vi "Init.vi"(8 "error in (no error)":errorcluster, 10 "Connection String":string, 11 "Camera in":refnum<class "CameraI2COUSB.lvclass">) -> (0 "error out":errorcluster, 3 "Camera out":refnum<class "CameraI2COUSB.lvclass">)   [LabVIEW 2020, in "CameraI2COUSB.lvlib" / "CameraI2COUSB.lvclass"]
doc: "Inizialize camera object\n\n<b> ConnectionString:</b> String with parameters needed to connecting to camera. The parameters are separate by ::\nThe format is: <Vid>::<Pid>::<Device Index>::<Clock Rate>::<Provider Name>"
uses:
  CameraI2COUSB.lvclass
  Private/TypeDef/Init_FSMDate.ctl
  Private/TypeDef/Init_Step.ctl
  CameraI2COUSB.lvclass/CameraI2COUSB.ctl
  <vilib>/Utility/error.llb/Error Cluster From Error Code.vi
  <vilib>/Utility/LVClass/Get LV Class Default Value.vi
  <vilib>/ErrorRing/Error Ring.xnode
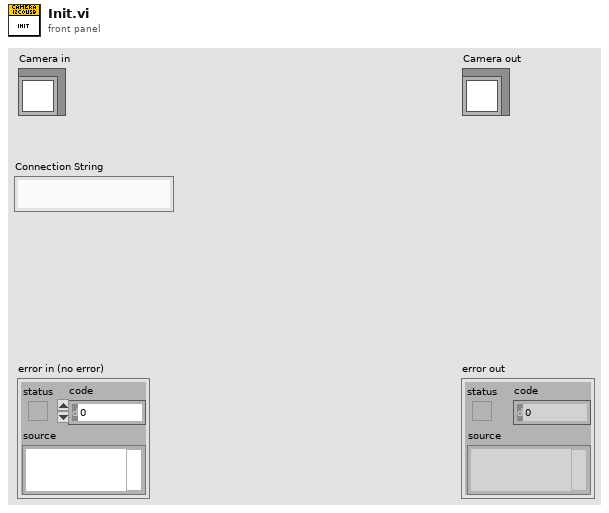
[diagram p1: front panel]
types:
  T1 = typedef "CameraI2COUSB.lvlib/CameraI2COUSB.lvclass/Init_FSMDate.ctl" = cluster{"States":T2[], "PrjctItemRef":refnum<vi>}
  T2 = typedef "CameraI2COUSB.lvlib/CameraI2COUSB.lvclass/Init_Step.ctl" = enum16{"AcquireConnPrms", "SetConfigParams", "CheckDriverFolder", "FindDriverClass", "LoadDriver", "Map Cmds to Registers", "Create Events"}
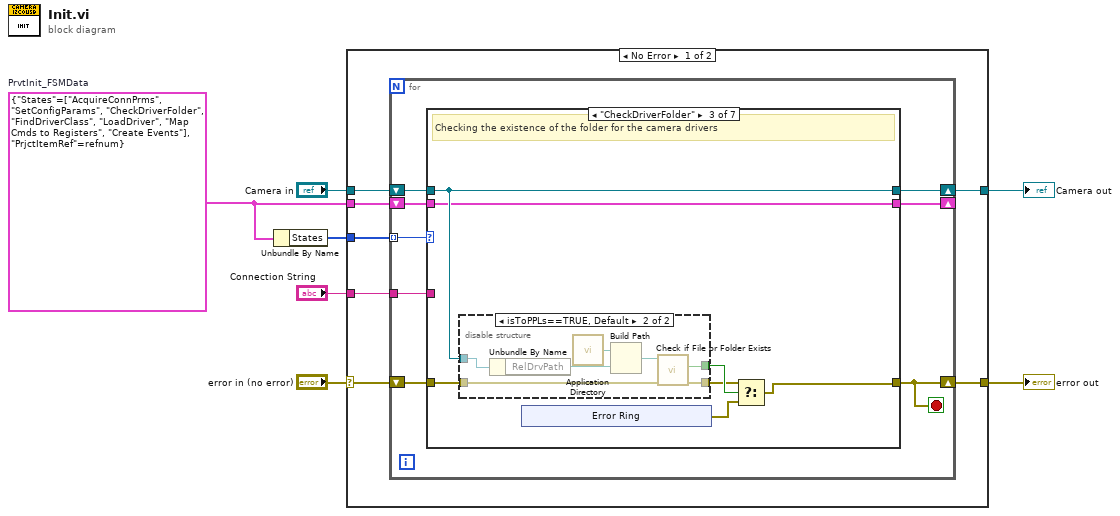
[diagram p0: block diagram]
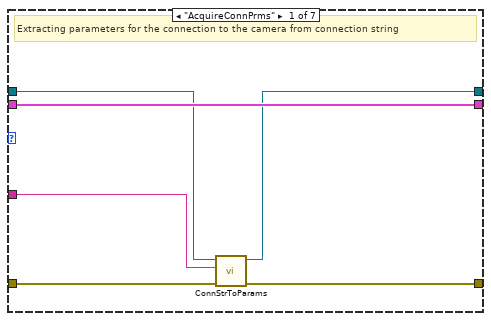
[diagram p2: hidden frame]
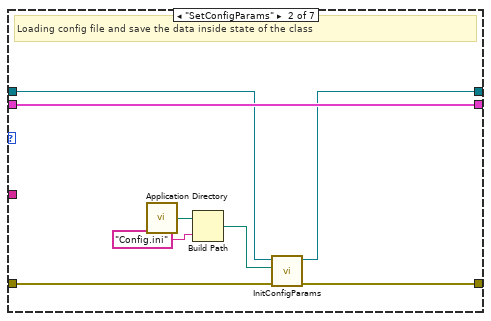
[diagram p3: hidden frame]
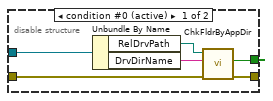
[diagram p4: hidden frame]
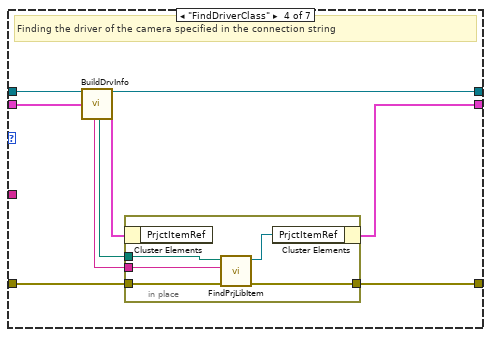
[diagram p5: hidden frame]
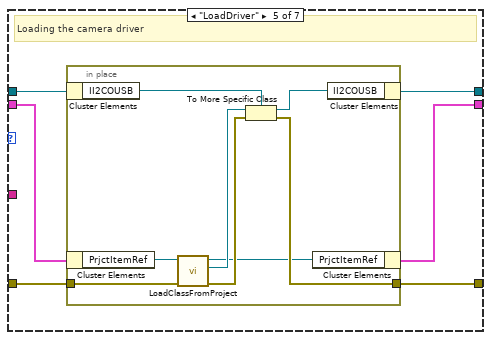
[diagram p6: hidden frame]
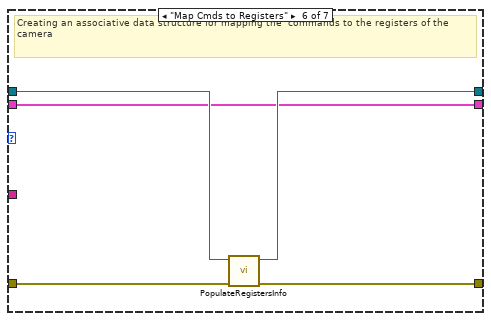
[diagram p7: hidden frame]
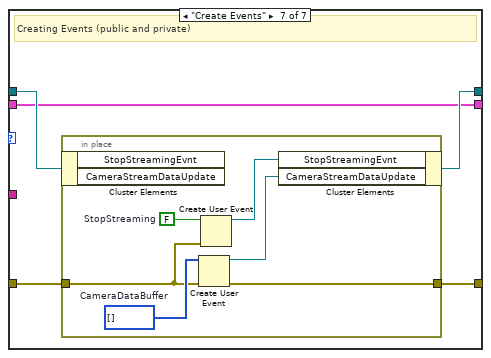
[diagram p8: hidden frame]
diagram:
  w6 = T1 {"States"=[enum."AcquireConnPrms", enum."SetConfigParams", enum."CheckDriverFolder", enum."FindDriverClass", enum."LoadDriver", enum."Map Cmds to Registers", enum."Create Events"], "PrjctItemRef"=refnum}  # PrvtInit_FSMData
  n1 = Unbundle By Name(w6) -> ("States"=w7:T2[])
  n2 = case shown="No Error" "error in (no error)" {
    selector: "error in (no error)" -> [w11 w106]
    tunnel: [w8 w106] -> w1
    tunnel: [w13 w105] -> w5
    tunnel: "Camera in" -> [w14 w105]
    tunnel: "Connection String" -> [w12 _]
    tunnel: w6 -> [w10 _]
    tunnel: w7 -> [w9 _]
    frame No Error {
      n3 = for {
        shift-right: [w19] -> w13
        shift-left: w14 -> [w20]
        tunnel: w12 -> [w22]
        shift-right: [w15] -> w8
        shift-left: w11 -> [w21]
        shift-right: [w17] -> _
        shift-left: w10 -> [w18]
        tunnel: w9 -> [w16] mode=indexing
        stop <- w15 stop-if-true
        n4 = case shown="\"CheckDriverFolder\"" w16 {
          tunnel: w22 -> [w28 _ _ _ _ _ _]
          tunnel: w21 -> [w25 w29 w43 w63 w80 w92 w95]
          tunnel: [w24 w35 w37 w62 w77 w90 w94] -> w15
          tunnel: w20 -> [w26 w33 w42 w67 w79 w93 w98]
          tunnel: [w23 w34 w42 w66 w76 w91 w97] -> w19
          tunnel: w18 -> [w27 w36 w41 w69 w78 w89 w96]
          tunnel: [w27 w36 w41 w68 w75 w89 w96] -> w17
          frame "AcquireConnPrms" {
            # "Extracting parameters for the connection to the camera from connection string"
            n5 = call "ConnStrToParams.vi"("error in (no error)"=w25, "Connection String"=w28, "Camera in"=w26) -> ("error out"=w24:errorcluster, "Camera out"=w23:refnum<class "CameraI2COUSB.lvclass">)  [unwired: 7 in]
          }
          frame "SetConfigParams" {
            # "Loading config file and save the data inside state of the class"
            n6 = call <vilib>:"Application Directory.vi"() -> ("Application Directory"=w30:path)
            n7 = Build Path(base path=w30, name or relative path="Config.ini") -> (appended path=w31:path)
            n8 = call "InitConfigParams.vi"("error in (no error)"=w29, "configuration file path"=w31, "Camera in"=w33) -> ("error out"=w35:errorcluster, "Camera out"=w34:refnum<class "CameraI2COUSB.lvclass">)  [unwired: 7 in]
          }
          frame "CheckDriverFolder" {
            # "Checking the existence of the folder for the camera drivers"
            n9 = disable-structure shown="isToPPLs==TRUE, Default" {
              disable-tunnel: w43 -> [w54 w59]
              disable-tunnel: [w49 w58] -> w38
              disable-tunnel: w42 -> [w53 w56]
              disable-tunnel: [w50 w57] -> w39
              frame condition #0 (active) {
                n10 = Unbundle By Name(w53) -> ("RelDrvPath"=w52:path, "DrvDirName"=w51:string)
                n11 = call "ChkFldrByAppDir.vi"("error in (no error)"=w54, "Folder Name"=w51, "Rel. Path"=w52) -> ("error out"=w49:errorcluster, "file or folder exists?"=w50:bool)  [unwired: 7 in]
              }
              frame condition #1 {
                n12 = Unbundle By Name(w56) -> ("RelDrvPath"=w55:path)
                n13 = call <vilib>:"Application Directory.vi"() -> ("Application Directory"=w60:path)
                n14 = Build Path(base path=w60, name or relative path=w55) -> (appended path=w61:path)
                n15 = call <vilib>:"Check if File or Folder Exists.vi"("error in (no error)"=w59, "path"=w61) -> ("error out"=w58:errorcluster, "file or folder exists?"=w57:bool)  [unwired: 7 in, 1 out]
              }
            }
            n16 = xnode "Error Ring"() -> ("error out"=w40:errorcluster)
            n17 = Select(t=w38, s=w39, f=w40) -> (s? t:f=w37:errorcluster)
          }
          frame "FindDriverClass" {
            # "Finding the driver of the camera specified in the connection string"
            n18 = call "BuildDrvInfo.vi"("Camera in"=w67) -> ("Camera out"=w66:refnum<class "CameraI2COUSB.lvclass">, "Lib Path"=w65:path, "Class Name"=w64:string)  [unwired: 16 in]
            n19 = in-place {
              in-place-border: w65 -> [w73]
              in-place-border: w64 -> [w72]
              in-place-border: w63 -> [w71]
              in-place-border: [w70] -> w62
              n20 = in-place-cluster #1(w69) -> ()  [unwired: 1 out]
              n21 = call "FindPrjLibItem.vi"("error in (no error)"=w71, "Item Name"=w72, "Lib Path"=w73) -> ("error out"=w70:errorcluster, "ProjectItem Refnum"=w74:refnum<vi>)  [unwired: 7 in]
              n22 = in-place-cluster #1("PrjctItemRef"=w74) -> (w68:T1)
            }
          }
          frame "LoadDriver" {
            # "Loading the camera driver"
            n23 = in-place {
              in-place-border: w80 -> [w87]
              in-place-border: [w83] -> w77
              n24 = in-place-cluster #2(w79) -> ("II2COUSB"=w88:refnum<class "II2COUSB.lvclass">)
              n25 = in-place-cluster #3(w78) -> ("PrjctItemRef"=w86:refnum<vi>)
              n26 = call "LoadClassFromProject.vi"("error in (no error)"=w87, "PrjctItemRef"=w86) -> ("error out"=w82:errorcluster, "object"=w85:refnum<class>, "PrjctItemRef"=w81:refnum<vi>)  [unwired: 7 in]
              n27 = To More Specific Class(target class=w88, reference=w85, error in=w82) -> (specific class reference=w84:refnum<class "II2COUSB.lvclass">, error out=w83:errorcluster)
              n28 = in-place-cluster #3("PrjctItemRef"=w81) -> (w75:T1)
              n29 = in-place-cluster #2("II2COUSB"=w84) -> (w76:refnum<class "CameraI2COUSB.lvclass">)
            }
          }
          frame "Map Cmds to Registers" {
            # "Creating an associative data structure for mapping the  commands to the registers of the camera"
            n30 = call "PopulateRegistersInfo.vi"("error in (no error)"=w92, "Camera in"=w93) -> ("error out"=w90:errorcluster, "Camera out"=w91:refnum<class "CameraI2COUSB.lvclass">)  [unwired: 8 in]
          }
          frame "Create Events" {
            # "Creating Events (public and private)"
            n31 = in-place {
              in-place-border: w95 -> [w101]
              in-place-border: [w103] -> w94
              w102 = FALSE  # StopStreaming
              w104 = u8[] []  # CameraDataBuffer
              n32 = in-place-cluster #4(w98) -> ()  [unwired: 2 out]
              n33 = Create User Event(user event datatype=w104, error in=w101) -> (user event=w100:refnum<user-event>, error out=w103:errorcluster)
              n34 = Create User Event(user event datatype=w102, error in=w101) -> (user event=w99:refnum<user-event>)  [unwired: 1 out]
              n35 = in-place-cluster #4("StopStreamingEvnt"=w99, "CameraStreamDataUpdate"=w100) -> (w97:refnum<class "CameraI2COUSB.lvclass">)
            }
          }
        }
      }
    }
    frame Error {
    }
  }
  "error out" <- w1
  "Camera out" <- w5
